vi "OPC UA Server.vi"() -> ()   [LabVIEW 2017]
uses:
  <vilib>/OPCUA/NI OPC UA Server.lvlib
panel:
  out "Item Path":string="Process Data.Temperature"
  in  "Stop Button":bool
  out "Server Endpoint URL":string="opc.tcp://PORS-3650:49580"
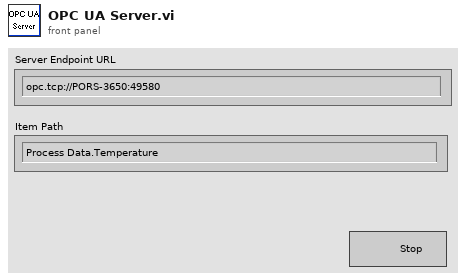
[diagram p1: front panel]
types:
  T1 = cluster{"name":string, "data type":u16, "access level":u16, "description":string}
  T2 = typedef "OPC UA Server Refnum.ctl" = refnum<k21>
  T3 = typedef "NodeId.ctl" = string
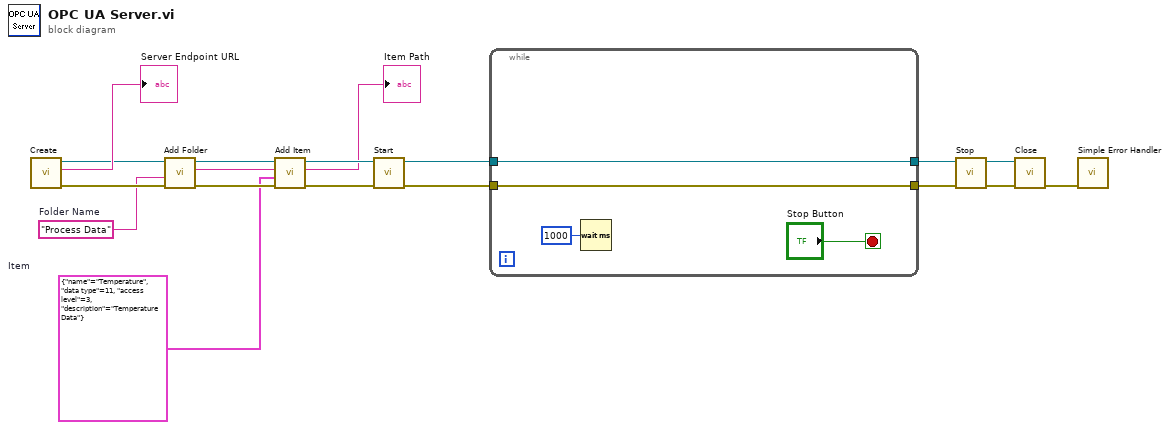
[diagram p0: block diagram]
diagram:
  w5 = T1 {"name"="Temperature", "data type"=11, "access level"=3, "description"="Temperature Data"}  # Item
  w12 = "Process Data"  # Folder Name
  n1 = call <vilib>:"Create.vi"() -> ("error out"=w18:errorcluster, "server endpoint URL"=→"Server Endpoint URL":string, "OPC UA server refnum out"=w11:T2)  [unwired: 9 in]
  n2 = call <vilib>:"Add Folder.vi"("error in (no error)"=w18, "folder name"=w12, "OPC UA server refnum in"=w11) -> ("error out"=w17:errorcluster, "folder node ID"=w6:T3, "OPC UA server refnum out"=w10:T2)  [unwired: 5 in]
  n3 = call <vilib>:"Add Item.vi"("error in (no error)"=w17, "item"=w5, "parent folder node ID"=w6, "OPC UA server refnum in"=w10) -> ("error out"=w7:errorcluster, "item node ID"=→"Item Path":T3, "OPC UA server refnum out"=w8:T2)  [unwired: 3 in, 1 out]
  n4 = call <vilib>:"Start.vi"("error in (no error)"=w7, "OPC UA server refnum in"=w8) -> ("error out"=w16:errorcluster, "OPC UA server refnum out"=w9:T2)  [unwired: 7 in, 1 out]
  n5 = while {
    tunnel: w16 -> [w19]
    tunnel: w9 -> [w20]
    tunnel: [w20] -> w2
    tunnel: [w19] -> w1
    stop <- "Stop Button" stop-if-true
    n6 = Wait (ms)(milliseconds to wait=u32 1000) -> ()  [unwired: 1 out]
  }
  n7 = call <vilib>:"Stop.vi"("error in (no error)"=w1, "OPC UA server refnum in"=w2) -> ("error out"=w14:errorcluster, "OPC UA server refnum out"=w4:T2)  [unwired: 8 in]
  n8 = call <vilib>:"Close.vi"("error in (no error)"=w14, "OPC UA server refnum in"=w4) -> ("error out"=w13:errorcluster)  [unwired: 9 in]
  n9 = call <vilib>:"Simple Error Handler.vi"("error in (no error)"=w13) -> ()  [unwired: 4 in, 5 out]
